vi "WallAllignment.vi"(7 "Score cutoff":dbl, 8 "error in":errorcluster, 9 "Color Components":T2={"Hue"={110.0, 142.0}, "Sat"={138.0, 255.0}, "Val"={139.0, 198.0}} {"Val" scale=0.0..255.0; "Sat" scale=0.0..255.0; "Hue" scale=0.0..255.0 scale format="%#_3g"}, 10 "Color System":u16(ring)=2 items=["RGB", "HSL", "HSV", "HSI"], 11 "Image":T1) -> (0 "error out":errorcluster, 3 "Image out":T1)   [LabVIEW 2013]
doc: "Determines if the goal is hot or not and returns an enum to indicate this. Also returns the calculated distance to the goal."
uses:
  <vilib>/vision/Image Controls.llb/IMAQ Image.ctl
  Example_Code/Ultrasonic/SonarAction.ctl
  <vilib>/Rock Robotics/WPI/RobotDrive/WPI_RobotDriveGetSetRefNum.vi
  <vilib>/addons/control/pid/pid.llb/PID (DBL).vi
  <vilib>/Rock Robotics/WPI/RobotDrive/WPI_RobotDriveArcadeDrive_Standard(NoSaturation).vi
  <vilib>/addons/control/pid/NI_PID_pid.lvlib
panel:
  in  "Camera Type":enum16{"206", "1011", "1013"}(ring)=enum."1013"
  in  "Area Size Limit %":dbl=0.06 format="%#_13g"
  out "Mask":T1(plugin-control)
  out "Image":T1(plugin-control)
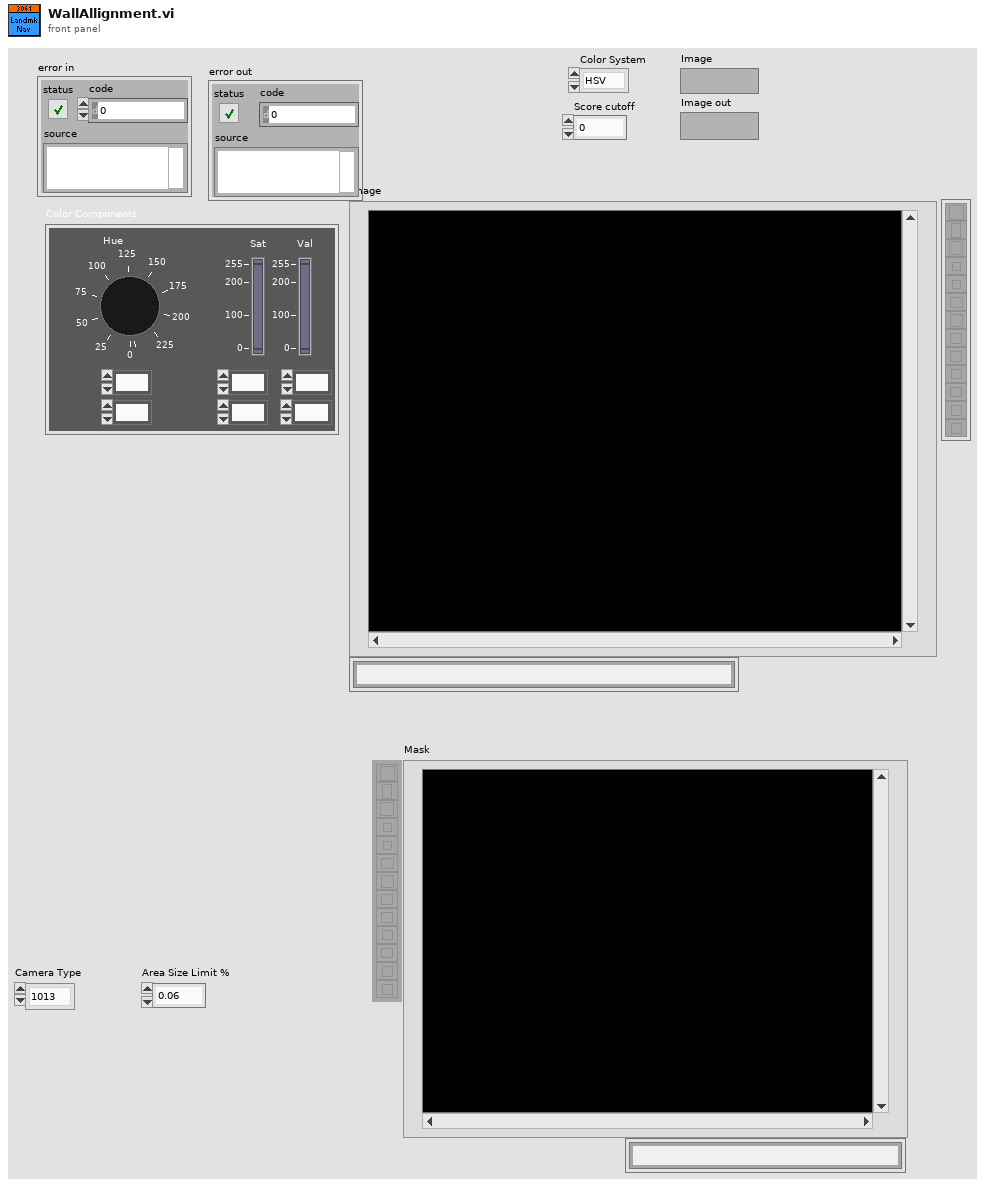
[diagram p1: front panel]
types:
  T1 = typedef "IMAQ Image.ctl" = refnum<image>
  T2 = cluster{"Hue":cluster{dbl, dbl}, "Sat":cluster{dbl, dbl}, "Val":cluster{dbl, dbl}}
  T3 = typedef "SonarAction.ctl" = enum16{"Init", "ReadValue", "Disable"}
  T4 = cluster{"Horizontal":bool, "Aspect Score":dbl, "Rect Score":dbl, cluster{"Left":dbl, "Top":dbl, "Right":dbl, "Bottom":dbl}, "Equiv H":dbl, "Equiv V":dbl}[]
  T5 = typedef "TargetType.ctl" = enum16{"Not Hot", "Hot"}
  T6 = cluster{"Scores":cluster{"Total":dbl, "Left":dbl, "Right":dbl, "Ratio":dbl, "Vertical":dbl, "index":i32, "State":T5}, "Verticals":cluster{"Horizontal?":bool, "Aspect Score":dbl, "Rect Score":dbl, cluster{"Left":dbl, "Top":dbl, "Right":dbl, "Bottom":dbl}, "Equiv H":dbl, "Equiv V":dbl}, "Horizontals":cluster{"Horizontal?":bool, "Aspect Score":dbl, "Rect Score":dbl, cluster{"Left":dbl, "Top":dbl, "Right":dbl, "Bottom":dbl}, "Equiv H":dbl, "Equiv V":dbl}, "Validated":bool}[]
  T7 = cluster{"Distance (ft)":dbl, "Target Center (-1 to 1)":cluster{"X":dbl, "Y":dbl}, bool, "State":T5, "Target Center (Angles)":cluster{dbl, dbl}, "Center Displacement (ft)":dbl}[]
  T8 = typedef "WPI_RobotDriveDevRef.ctl" = cluster{"DevStatus":errorcluster, "Motors[]":T9[], "Square Inputs":bool, "Max Output":dbl, "Isochronous":bool}
  T9 = typedef "WPI_MotorControlDeviceRef.ctl" = cluster{"DeviceStatus":errorcluster, "Type":enum16{"PWM", "CAN"}, "PWM":cluster{"Digital Module":T10, "PWM Channel":T11, "DeadBand":T12}, "CAN":cluster{"Device Number":u8, "Control Mode":T13, "Semaphore":T14, "Max Vout":dbl}, "Invert":bool, "TransformRef":T15, "InvTransformRef":T15}
  T10 = typedef "FPGA_TypedefDigitalModule.ctl" = enum16{"Digital Module 1", "Digital Module 2"}
  T11 = typedef "FPGA_DIOPWMChannel.ctl" = enum8{"PWM 1", "PWM 2", "PWM 3", "PWM 4", "PWM 5", "PWM 6", "PWM 7", "PWM 8", "PWM 9", "PWM 10", "Invalid"}
  T12 = typedef "WPI_PWMDeadband.ctl" = cluster{"Name":string, "maxPositivePwm":i32, "minPositivePwm":i32, "centerPwm":i32, "maxNegativePwm":i32, "minNegativePwm":i32, "angularRange":u16}
  T13 = typedef "WPI_CANJaguar_ControlMode.ctl" = enum8{"Percent VBus", "Current", "Speed", "Position", "Voltage"}
  T14 = typedef "Semaphore RefNum" = refnum<k1>
  T15 = typedef "WPI_PWMTransform_ConPane.ctl" = refnum<vi>
  T16 = cluster{"Distance (ft)":dbl, "Target Center (-1 to 1)":cluster{"X":dbl, "Y":dbl}, bool, "State":T5, "Target Center (Angles)":cluster{dbl, dbl}, "Center Displacement (ft)":dbl}
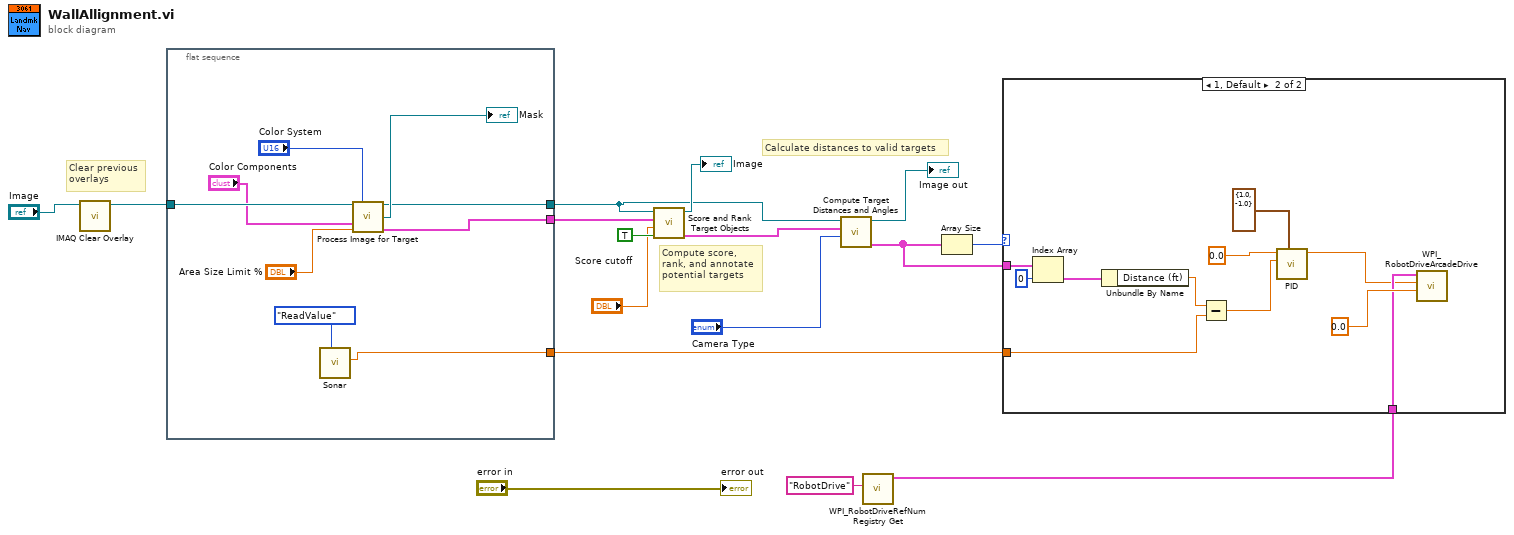
[diagram p0: block diagram]
diagram:
  # "Calculate distances to valid targets"
  # "Clear previous\noverlays"
  # "Compute score,\nrank, and annotate\npotential targets"
  n1 = call "IMAQ Clear Overlay"("Image"="Image") -> ("Image Out"=w9:T1)  [unwired: 9 in, 1 out]
  n2 = flat-sequence {
    tunnel: [w23] -> w3
    tunnel: [w22] -> w15
    tunnel: w9 -> [w20]
    tunnel: [w18] -> w4
    frame #0 {
      n3 = call "Sonar.vi"("Action"=SonarAction."ReadValue") -> ("distance"=w18:dbl)  [unwired: 9 in, 1 out]
      n4 = call "Process Image for Target.vi"("Src Image"=w20, "Color Mode"="Color System", "Color Components"="Color Components", "Area Cutoff %"="Area Size Limit %") -> ("Src Image Out"=w23:T1, "Threshold"=→"Mask":T1, "Particles"=w22:T4)  [unwired: 9 in]
    }
  }
  n5 = call "Score and Rank Target Objects.vi"("Annotate"=TRUE, "Score Limit"="Score cutoff", "Particles"=w15, "Image in"=w3) -> ("Target Info"=w10:T6, "Annotated Image"=→"Image":T1)  [unwired: 6 in]
  n6 = call "Compute Target Distances and Angles.vi"("Camera Type"="Camera Type", "Target Info"=w10, "Image in"=w3) -> ("Distances"=w5:T7, "Image out"=→"Image out":T1)  [unwired: 6 in, 1 out]
  n7 = call <vilib>:"WPI_RobotDriveRefNum Registry Get.vi"("refnum name"="RobotDrive") -> ("RobotDriveDevRef"=w1:T8)  [unwired: 9 in, 1 out]
  n8 = Array Size(array=w5) -> (size(s)=w6:i32)
  n9 = case shown="1, Default" w6 {
    tunnel: w5 -> [_ w36]
    tunnel: w4 -> [_ w29]
    tunnel: w1 -> [_ w27]
    frame 0 {
    }
    frame 1, Default {
      n10 = Index Array(array=w36, index=0) -> (element=w34:T16)
      n11 = Unbundle By Name(w34) -> ("Distance (ft)"=w33:dbl)
      n12 = Subtract(x=w33, y=w29) -> (x-y=w32:dbl)
      n13 = call-poly <vilib>:"PID.vi"("output range"=cluster{"output high":dbl, "output low":dbl} {"output high"=1.0, "output low"=-1.0}, "process variable"=w32, "setpoint"=0.0) -> ("output"=w26:dbl)  [unwired: 7 in, 1 out]
      n14 = call-poly <vilib>:"WPI_RobotDriveArcadeDrive.vi"("Y axis value"=0.0, "X axis value"=w26, "RobotDriveDevRef"=w27) -> ()  [unwired: 6 in, 3 out]
    }
  }
  "error out" <- "error in"
